vi "SWERVE_DRIVE_AQUIRE.vi"(6 "Pass_Through_Time":dbl=-1.0 format="%33.4f", 8 "GyroDevRef":T1={"DevStatus"={"status"=FALSE, "code"=0, "source"=""}, "Analog Channel"=enum."AI 1", "Gain (VoltsPerDegree/Second)"=0.0, "Gyro Type"=enum."Analog", "Handle"=0, "SPI Bus"=enum."Invalid", "Device Found"=FALSE, "Sample Rate"=1.0, "Calibrate On Open"=FALSE, "Offset"=0.0} {"Sample Rate" min=0.25 max=100.0 step=0.25}, 9 "in Swerve Module States":T6[](array[typedef]) {"Angle"."SIN" format="%13.4f"; "Angle"."COS" format="%13.4f"; "Angle"."VALUE" format="%13.4f"}, 10 "Swerve IO Reference":T7[](array[typedef]), 11 "in SWERVE_DRIVE_KINEMATICS":T17 {"SavedModuleStates"."Angle"."SIN" format="%13.4f"; "SavedModuleStates"."Angle"."COS" format="%13.4f"; "SavedModuleStates"."Angle"."VALUE" format="%13.4f"; "PrevCoR"."Y" format="%14.3f"; "PrevCoR"."X" format="%14.3f"; "Modules"."Y" format="%14.3f"; "Modules"."X" format="%14.3f"}) -> (0 "out Swerve Module Positions":T4[](array[typedef]) {"Angle"."SIN" format="%13.4f"; "Angle"."COS" format="%13.4f"; "Angle"."VALUE" format="%13.4f"}, 1 "out Swerve Module States":T6[](array[typedef]) {"Angle"."SIN" format="%13.4f"; "Angle"."COS" format="%13.4f"; "Angle"."VALUE" format="%13.4f"}, 2 "Gyro_Heading_Rad":dbl, 3 "Gyro_Continuous_Rad":dbl)   [LabVIEW 2019]
uses:
  <vilib>/Rock Robotics/WPI/ThirdParty/JAS_Junk/TrajLib/TypeDef/SWERVE_DRIVE_KINEMATICS.ctl
  <vilib>/Analysis/Matrix/Datatypes/RealMatrix.ctl
  <vilib>/Rock Robotics/WPI/ThirdParty/JAS_Junk/TrajLib/TypeDef/TRANSLATION2D.ctl
  <vilib>/Rock Robotics/WPI/ThirdParty/JAS_Junk/TrajLib/TypeDef/SWERVE_DRIVE_MODULE_STATE.ctl
  <vilib>/Rock Robotics/WPI/ThirdParty/JAS_Junk/TrajLib/TypeDef/ROTATION2D.ctl
  SWERVE_DRIVE_MODULE_TYPDEF.ctl
  <vilib>/Rock Robotics/WPI/MotorControl/WPI_MotorControlDeviceRef.ctl
  <vilib>/Rock Robotics/WPI/MotorControl/WPI_MotorControlType.ctl
  <vilib>/Rock Robotics/SystemInterfaces/DIO/FPGA_DIOPWMChannel.ctl
  <vilib>/Rock Robotics/WPI/PWM/WPI_PWMDeadband.ctl
  <vilib>/Rock Robotics/SystemInterfaces/DIO/FPGA_DIOChannel.ctl
  <vilib>/Rock Robotics/WPI/Encoder/WPI_EncoderDevRef.ctl
  <vilib>/Rock Robotics/SystemInterfaces/Encoder/FPGA_EncoderIdx.ctl
  <vilib>/Rock Robotics/SystemInterfaces/Counter/FPGA_CounterCtrSystemIndex.ctl
  <vilib>/Rock Robotics/WPI/Encoder/WPI_EncoderType.ctl
  <vilib>/Rock Robotics/WPI/ThirdParty/JAS_Junk/TrajLib/TypeDef/SWERVE_DRIVE_MODULE_POSITION.ctl
  <vilib>/Rock Robotics/WPI/Gyro/WPI_GyroDevRef.ctl
  <vilib>/Rock Robotics/SystemInterfaces/AI/FPGA_AIChannel.ctl
  <vilib>/Rock Robotics/SystemInterfaces/spilib/spi_bus.ctl
  Robot Global Data.vi
  <vilib>/Rock Robotics/WPI/ThirdParty/JAS_Junk/TrajLib/Trajectory_Library.lvlib
  Secret_Control_Library_Protected/Secret_Control_Library_Protected.lvlib
  <vilib>/Analysis/Matrix/NI_Matrix.lvlib
panel:
  # "Analog"
  # "XRS"
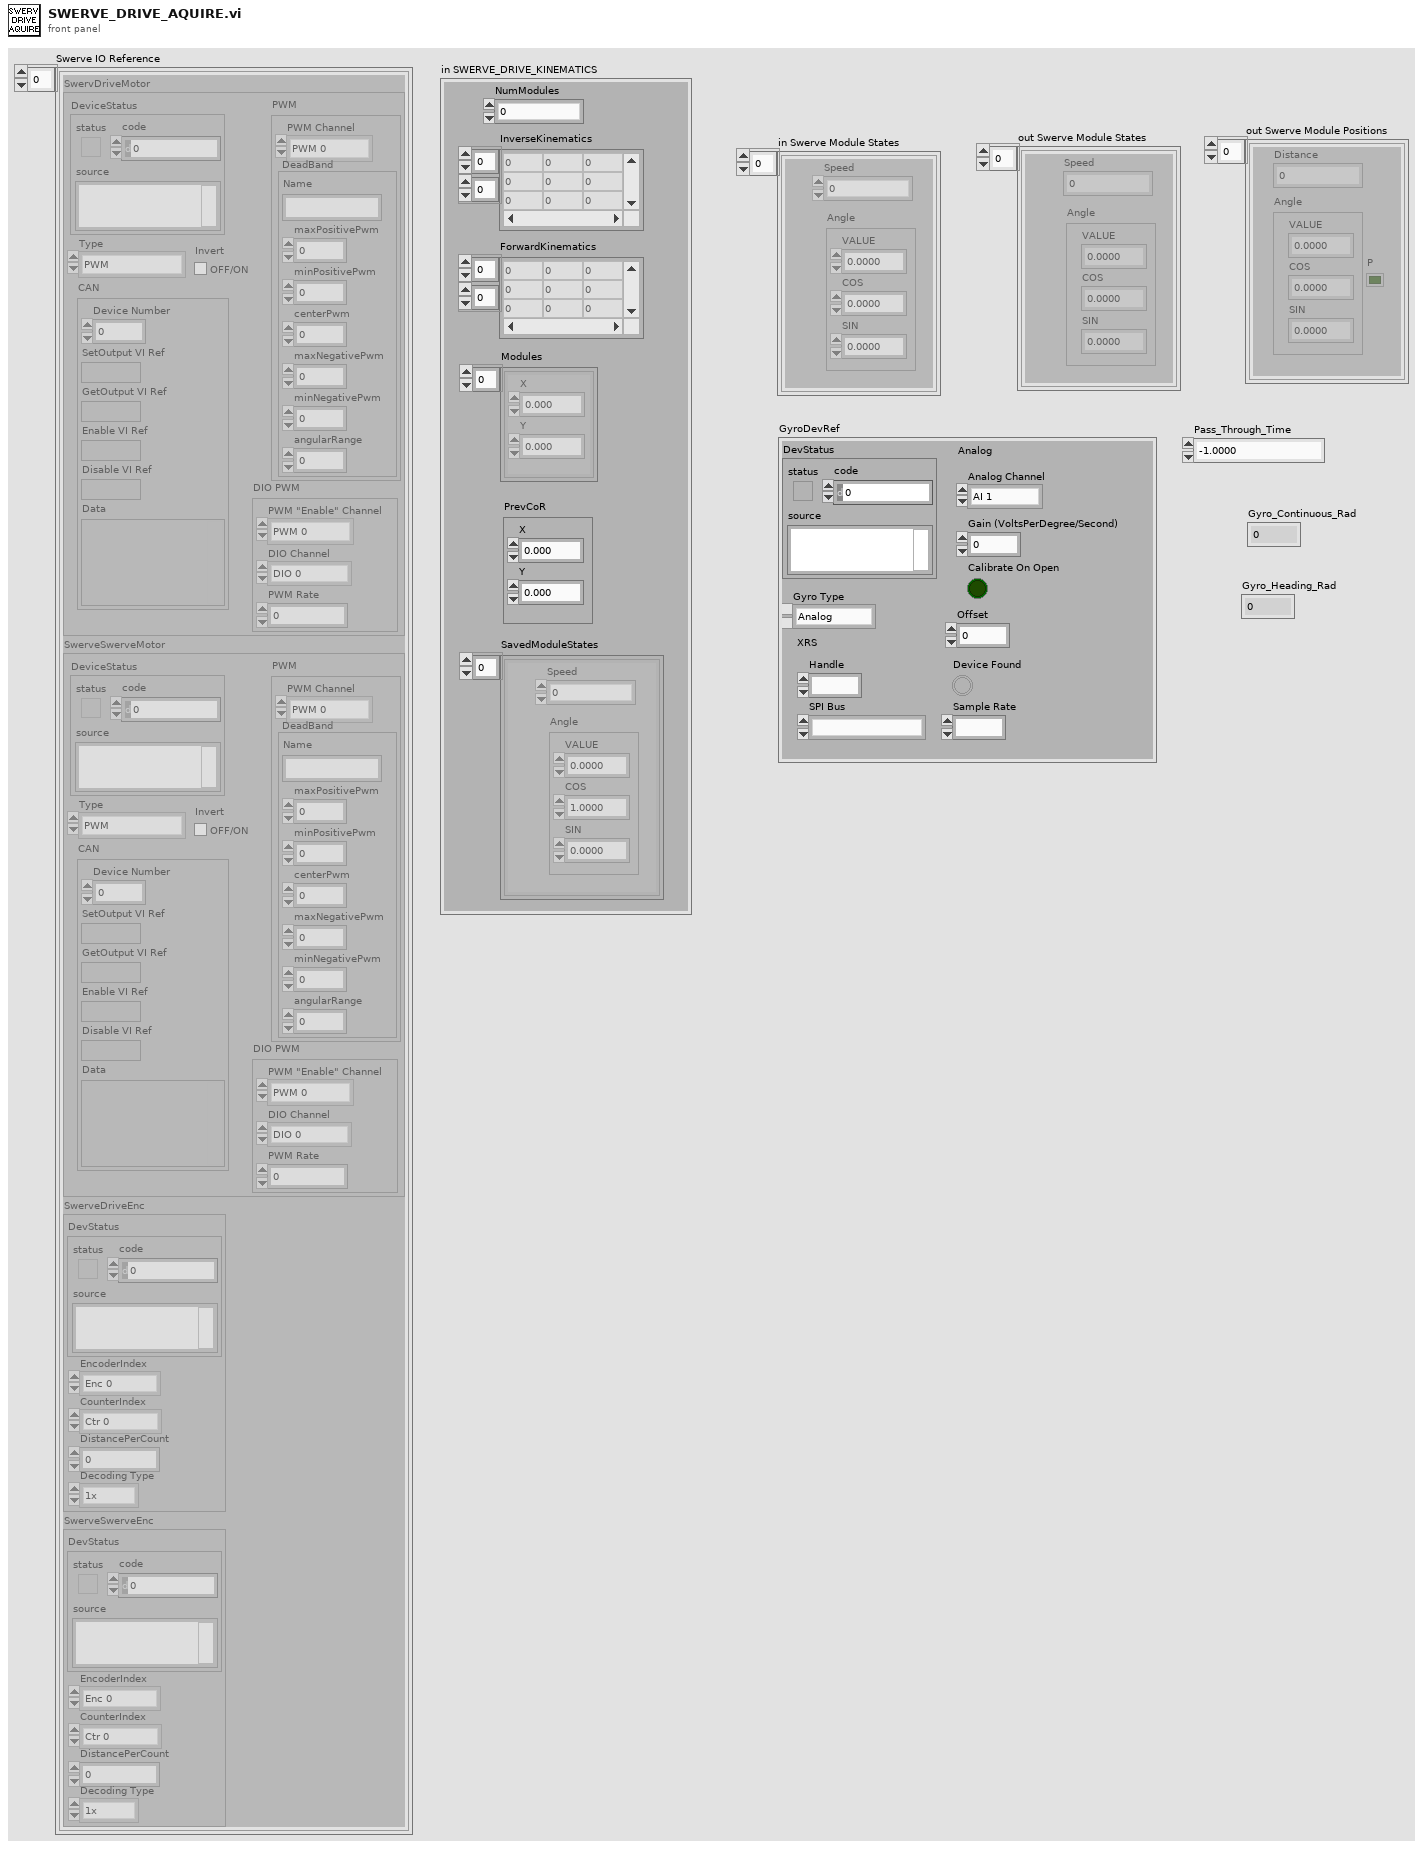
[diagram p1: front panel]
types:
  T1 = typedef "WPI_GyroDevRef.ctl" = cluster{"DevStatus":errorcluster, "Analog Channel":T2, "Gain (VoltsPerDegree/Second)":dbl, "Gyro Type":enum16{"Analog", "XRS450"}, "Handle":i32, "SPI Bus":T3, "Device Found":bool, "Sample Rate":dbl, "Calibrate On Open":bool, "Offset":dbl}
  T2 = typedef "FPGA_AIChannel.ctl" = enum8{"AI 0", "AI 1", "AI 2", "AI 3", "AI MXP 0", "AI MXP 1", "AI MXP 2", "AI MXP 3", "Invalid"}
  T3 = typedef "spi_bus.ctl" = enum16{"SPI On-Board, CS0", "SPI On-Board, CS1", "SPI On-Board, CS2", "SPI On-Board, CS3", "SPI MXP", "Invalid"}
  T4 = typedef "Trajectory_Library.lvlib/SWERVE_DRIVE_MODULE_POSITION.ctl" = cluster{"Distance":dbl, "Angle":T5, "P":bool}
  T5 = typedef "Trajectory_Library.lvlib/ROTATION2D.ctl" = cluster{"VALUE":dbl, "COS":dbl, "SIN":dbl}
  T6 = typedef "Trajectory_Library.lvlib/SWERVE_DRIVE_MODULE_STATE.ctl" = cluster{"Speed":dbl, "Angle":T5}
  T7 = typedef "SWERVE_DRIVE_MODULE_TYPDEF.ctl" = cluster{"SwervDriveMotor":T8, "SwerveSwerveMotor":T8, "SwerveDriveEnc":T13, "SwerveSwerveEnc":T13}
  T8 = typedef "WPI_MotorControlDeviceRef.ctl" = cluster{"DeviceStatus":errorcluster, "Type":T9, "PWM":cluster{"PWM Channel":T10, "DeadBand":T11}, "CAN":cluster{"Device Number":u8, "SetOutput VI Ref":variant, "GetOutput VI Ref":variant, "Enable VI Ref":variant, "Disable VI Ref":variant, "Data":variant}, "Invert":bool, "DIO PWM":cluster{"PWM \"Enable\" Channel":T10, "DIOChannel":T12, "PWM Rate":dbl}}
  T9 = typedef "WPI_MotorControlType.ctl" = enum16{"PWM", "CAN", "DIO PWM"}
  T10 = typedef "FPGA_DIOPWMChannel.ctl" = enum8{"PWM 0", "PWM 1", "PWM 2", "PWM 3", "PWM 4", "PWM 5", "PWM 6", "PWM 7", "PWM 8", "PWM 9", "PWM MXP 0", "PWM MXP 1", "PWM MXP 2", "PWM MXP 3", "PWM MXP 4", "PWM MXP 5", "PWM MXP 6", "PWM MXP 7", "PWM MXP 8", "PWM MXP 9", "Invalid"}
  T11 = typedef "WPI_PWMDeadband.ctl" = cluster{"Name":string, "maxPositivePwm":i32, "minPositivePwm":i32, "centerPwm":i32, "maxNegativePwm":i32, "minNegativePwm":i32, "angularRange":u16}
  T12 = typedef "FPGA_DIOChannel.ctl" = enum8{"DIO 0", "DIO 1", "DIO 2", "DIO 3", "DIO 4", "DIO 5", "DIO 6", "DIO 7", "DIO 8", "DIO 9", "DIO MXP 0", "DIO MXP 1", "DIO MXP 2", "DIO MXP 3", "DIO MXP 4", "DIO MXP 5", "DIO MXP 6", "DIO MXP 7", "DIO MXP 8", "DIO MXP 9", "DIO MXP 10", "DIO MXP 11", "DIO MXP 12", "DIO MXP 13", "DIO MXP 14", "DIO MXP 15", "SPI Port CS1", "SPI Port CS2", "SPI Port CS3", "SPI Port MISO", "SPI Port MOSI", "Invalid"}
  T13 = typedef "WPI_EncoderDevRef.ctl" = cluster{"DevStatus":errorcluster, "EncoderIndex":T14, "CounterIndex":T15, "DistancePerCount":dbl, "Decoding Type":T16}
  T14 = typedef "FPGA_EncoderIdx.ctl" = enum8{"Enc 0", "Enc 1", "Enc 2", "Enc 3", "Enc 4", "Enc 5", "Enc 6", "Enc 7", "Invalid"}
  T15 = typedef "FPGA_CounterCtrSystemIndex.ctl" = enum8{"Ctr 0", "Ctr 1", "Ctr 2", "Ctr 3", "Ctr 4", "Ctr 5", "Ctr 6", "Ctr 7", "Invalid"}
  T16 = typedef "WPI_EncoderType.ctl" = enum16{"1x", "2x", "4x"}
  T17 = typedef "Trajectory_Library.lvlib/SWERVE_DRIVE_KINEMATICS.ctl" = cluster{"NumModules":i32, "InverseKinematics":T18, "ForwardKinematics":T18, "Modules":T19[], "PrevCoR":T19, "SavedModuleStates":T6[]}
  T18 = typedef "NI_Matrix.lvlib/RealMatrix.ctl" = dbl[][]
  T19 = typedef "Trajectory_Library.lvlib/TRANSLATION2D.ctl" = cluster{"X":dbl, "Y":dbl}
  T20 = typedef "Trajectory_Library.lvlib/CHASSIS_SPEEDS.ctl" = cluster{"vX":dbl, "vY":dbl, "vOmega":dbl}
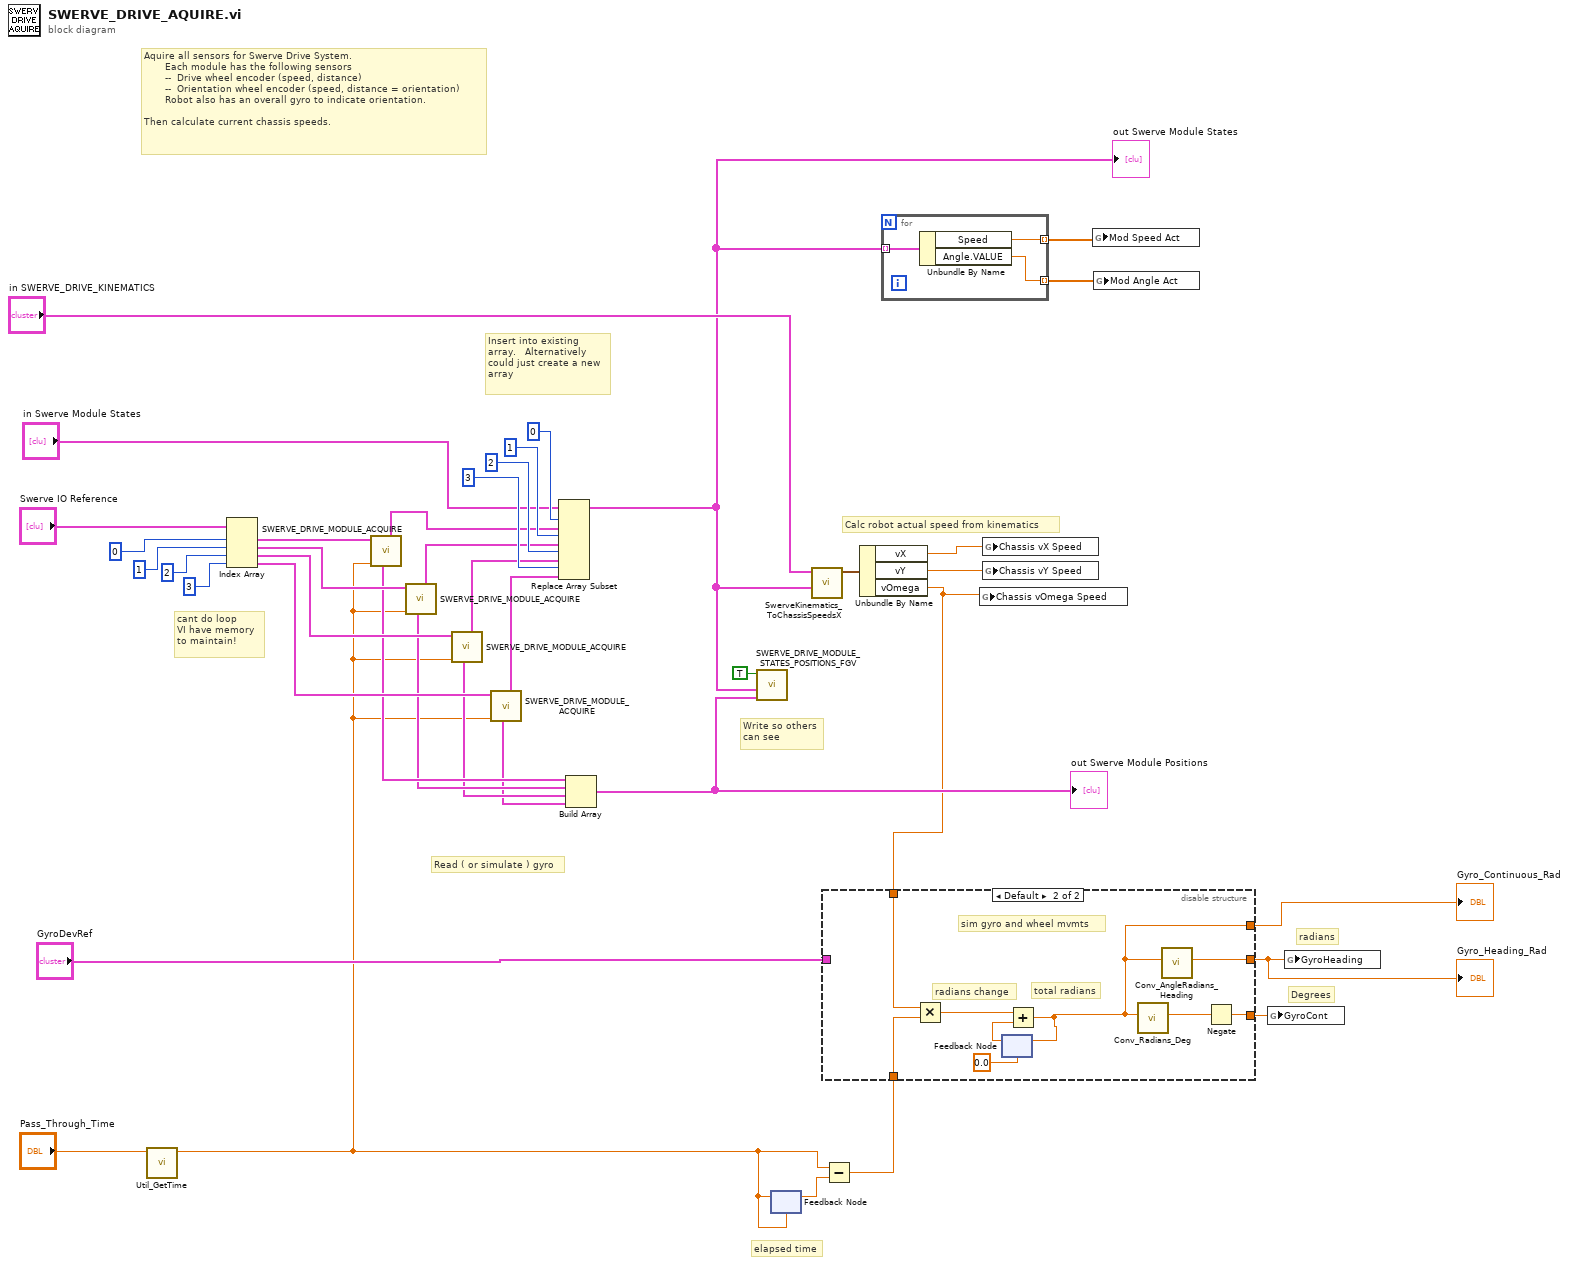
[diagram p0: block diagram]
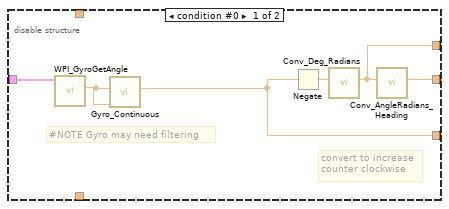
[diagram p2: hidden frame]
diagram:
  # "Read ( or simulate ) gyro"
  # "elapsed time"
  # "Degrees"
  # "radians"
  # "Aquire all sensors for Swerve Drive System.\n       Each module has the following sensors\n       --  Drive wheel encoder (speed, distance)\n       --  Orientation wheel encoder (speed, distance = orientation)\n       Robot also has an overall gyro to indicate orientation.\n\nThen calculate current chassis speeds."
  # "Insert into existing\narray.   Alternatively\ncould just create a new\narray"
  # "Calc robot actual speed from kinematics"
  # "Write so others\ncan see"
  # "cant do loop\nVI have memory\nto maintain!"
  n1 = call <vilib>:"Util_GetTime.vi"("Pass_Through_Time"="Pass_Through_Time") -> ("FPGA_Time_Seconds"=w4:dbl)  [unwired: 9 in, 1 out]
  n2 = Index Array(array="Swerve IO Reference", index #1=0 ("index"), index #2=1 ("index"), index #3=2 ("index"), index #4=3 ("index")) -> (element #1=w23:T7, element #2=w24:T7, element #3=w25:T7, element #4=w33:T7)
  n3 = call "SWERVE_DRIVE_MODULE_ACQUIRE.vi"("Pass_Through_Time"=w4, "Swerve Module TypDef"=w23) -> ("Swerve Module State"=w19:T6, "SWERVE DRIVE MODULE POSITION"=w17:T4)  [unwired: 3 in, 5 out]
  n4 = call "SWERVE_DRIVE_MODULE_ACQUIRE.vi"("Pass_Through_Time"=w4, "Swerve Module TypDef"=w24) -> ("Swerve Module State"=w22:T6, "SWERVE DRIVE MODULE POSITION"=w16:T4)  [unwired: 3 in, 5 out]
  n5 = call "SWERVE_DRIVE_MODULE_ACQUIRE.vi"("Pass_Through_Time"=w4, "Swerve Module TypDef"=w25) -> ("Swerve Module State"=w21:T6, "SWERVE DRIVE MODULE POSITION"=w15:T4)  [unwired: 3 in, 5 out]
  n6 = call "SWERVE_DRIVE_MODULE_ACQUIRE.vi"("Pass_Through_Time"=w4, "Swerve Module TypDef"=w33) -> ("Swerve Module State"=w34:T6, "SWERVE DRIVE MODULE POSITION"=w14:T4)  [unwired: 3 in, 5 out]
  n7 = Replace Array Subset(array="in Swerve Module States", new element #1=w19, index #1=0 ("index"), new element #2=w22, index #2=1 ("index"), new element #3=w21, index #3=2 ("index"), new element #4=w34, index #4=3 ("index")) -> (w1:T6[])
  "out Swerve Module States" <- w1
  n8 = Build Array(w17, w16, w15, w14) -> (w13:T4[])
  "out Swerve Module Positions" <- w13
  n9 = call "SWERVE_DRIVE_MODULE_STATES_POSITIONS_FGV.vi"("in Current Module Positions"=w13, "in Current Module States"=w1, "WRITE"=TRUE) -> ()  [unwired: 7 in, 2 out]
  n10 = feedback #1(w4) -> (w8:dbl)
  n11 = feedback-in #1(w4) -> ()
  n12 = call <vilib>:"SwerveKinematics_ToChassisSpeedsX.vi"("WheelStates"=w1, "in SWERVE_DRIVE_KINEMATICS"="in SWERVE_DRIVE_KINEMATICS") -> ("Chassis Speed"=w40:T20)  [unwired: 9 in]
  n13 = Subtract(x=w4, y=w8) -> (x-y=w7:dbl)
  n14 = Unbundle By Name(w40) -> ("vX"=w31:dbl, "vY"=w32:dbl, "vOmega"=w9:dbl)
  n15 = disable-structure shown="Default" {
    disable-tunnel: [w45 w52] -> w11
    disable-tunnel: [w43 w51] -> w12
    disable-tunnel: "GyroDevRef" -> [w42 _]
    disable-tunnel: w9 -> [_ w50]
    disable-tunnel: w7 -> [_ w48]
    disable-tunnel: [w41 w47] -> w5
    frame condition #0 {
      # "#NOTE Gyro may need filtering"
      # "convert to increase\ncounter clockwise"
      n16 = call <vilib>:"WPI_GyroGetAngle.vi"("GyroDevRef"=w42) -> ("Angle"=w44:dbl)  [unwired: 6 in, 4 out]
      n17 = call "Gyro_Continuous.vi"("GyroInitial"=w44, "GyroInput"=w44) -> ("GyroContinuous"=w43:dbl)  [unwired: 9 in]
      n18 = Negate(x=w43) -> (-x=w46:dbl)
      n19 = call <vilib>:"Conv_Deg_Radians.vi"("Degress"=w46) -> ("Radians"=w41:dbl)  [unwired: 10 in]
      n20 = call <vilib>:"Conv_AngleRadians_Heading.vi"("Radians"=w41) -> ("Heading"=w45:dbl)  [unwired: 10 in]
    }
    frame condition #1 (active) {
      # "total radians"
      # "radians change"
      # "sim gyro and wheel mvmts"
      n21 = Multiply(x=w50, y=w48) -> (x*y=w53:dbl)
      n22 = feedback #2(0.0) -> (w54:dbl)
      n23 = Add(x=w53, y=w54) -> (x+y=w47:dbl)
      n24 = feedback-in #2(w47) -> ()
      n25 = call <vilib>:"Conv_Radians_Deg.vi"("Radians"=w47) -> ("Degrees"=w49:dbl)  [unwired: 10 in]
      n26 = call <vilib>:"Conv_AngleRadians_Heading.vi"("Radians"=w47) -> ("Heading"=w52:dbl)  [unwired: 10 in]
      n27 = Negate(x=w49) -> (-x=w51:dbl)
    }
  }
  "Gyro_Heading_Rad" <- w11
  "Gyro_Continuous_Rad" <- w5
  n28 = for {
    tunnel: w1 -> [w58] mode=indexing
    tunnel: [w57] -> w2 mode=indexing
    tunnel: [w56] -> w3 mode=indexing
    n29 = Unbundle By Name(w58) -> ("Speed"=w56:dbl, "Angle.VALUE"=w57:dbl)
  }
  n30 = global write "Robot Global Data.vi" "Chassis vOmega Speed"(w9) -> ()
  n31 = global write "Robot Global Data.vi" "Chassis vX Speed"(w31) -> ()
  n32 = global write "Robot Global Data.vi" "Chassis vY Speed"(w32) -> ()
  n33 = global write "Robot Global Data.vi" "Mod Speed Act"(w3) -> ()
  n34 = global write "Robot Global Data.vi" "Mod Angle Act"(w2) -> ()
  n35 = global write "Robot Global Data.vi" "GyroCont"(w12) -> ()
  n36 = global write "Robot Global Data.vi" "GyroHeading"(w11) -> ()
